vi "校准中 (子VI).vi"(10 "校准按钮":refnum<vi>, 11 "曲线模型":refnum<vi>) -> ()   [LabVIEW 2016, in "斯坦道CODMn新电路板.lvlib"]
uses:
  <vilib>/ptbypt/NI_PtbyPt.lvlib
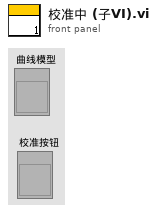
[diagram p1: front panel]
types:
  T1 = enum8{"Enabled", "Disabled", "Disabled and Grayed Out"}
  T2 = cluster{"时间标识":timestamp, "设备":string, "日志信息":string, "流程参数":string}
  T3 = cluster{"系统时间":timestamp, "工作状态":enum16{"空闲", "水样测试", "标样核查", "零点核查", "跨度核查", "空白测试", "平行样测试", "加标回收", "空白校准", "标样校准", "初始化（清洗）"}, "测量模式":enum16{"待机", "连续模式", "周期模式", "定点模式", "受控模式", "手动模式"}, "告警代码":u16, "故障代码":u16, "日志代码":u16, "软件版本":u16, "A":sgl, "B":sgl, "K":sgl, "当前滴定数":sgl, "T":sgl, "H":sgl, "id":u16, "flowid":u16, "量程":u16, "加热实时温度":sgl, "当前ORP值":sgl, "运行时间":sgl, "当前步骤剩余时间":sgl, "结束滴定数":sgl}
  T4 = enum16{"空闲", "水样测试", "标样核查", "零点核查", "跨度核查", "空白测试", "平行样测试", "加标回收", "空白校准", "标样校准", "初始化（清洗）"}
  T5 = cluster{"公式":cluster{"X^2":dbl, "X":dbl, "B":dbl}, "校准":cluster{"校准？":bool, "校准点1-5":u16, "校准浓度":dbl}}
  T6 = cluster{"标液浓度1":dbl, "测量吸光度1":dbl, "样品1启用":bool, "标液浓度2":dbl, "测量吸光度2":dbl, "样品2启用":bool, "标液浓度3":dbl, "测量吸光度3":dbl, "样品3启用":bool, "标液浓度4":dbl, "测量吸光度4":dbl, "样品4启用":bool, "标液浓度5":dbl, "测量吸光度5":dbl, "样品5启用":bool, "模型":enum32{"线性", "多项式"}, "method":enum16{"最小二乘", "最小绝对残差", "Bisquare"}, "精度":dbl, "XY图":cluster{"X Values":dbl[], "Y Values":dbl[]}[], "拟合公式":string, "r^2":dbl}
  T7 = cluster{"测量量程":dbl, "测量精度":dbl, "测量间隔":dbl, "消解温度":dbl, "消解时长":dbl, "空白校准时间":timestamp, "曲线截距":dbl, "曲线斜率":dbl, "测量检出限":dbl, "测量信号值":dbl, "线性相关系数":dbl, "二次多项式系数":dbl, "标样校准时间":timestamp, "稀释倍数":dbl, "三项式系数":dbl, "空白标定系数":dbl, "量程系数":dbl, "F0/ORPA":dbl, "F1/ORPB":dbl, "F2/ORPK":dbl, "F3":dbl, "F4":dbl, "F5":dbl, "F6":dbl, "F7":dbl, "X0/滴定数":dbl, "量程":dbl}
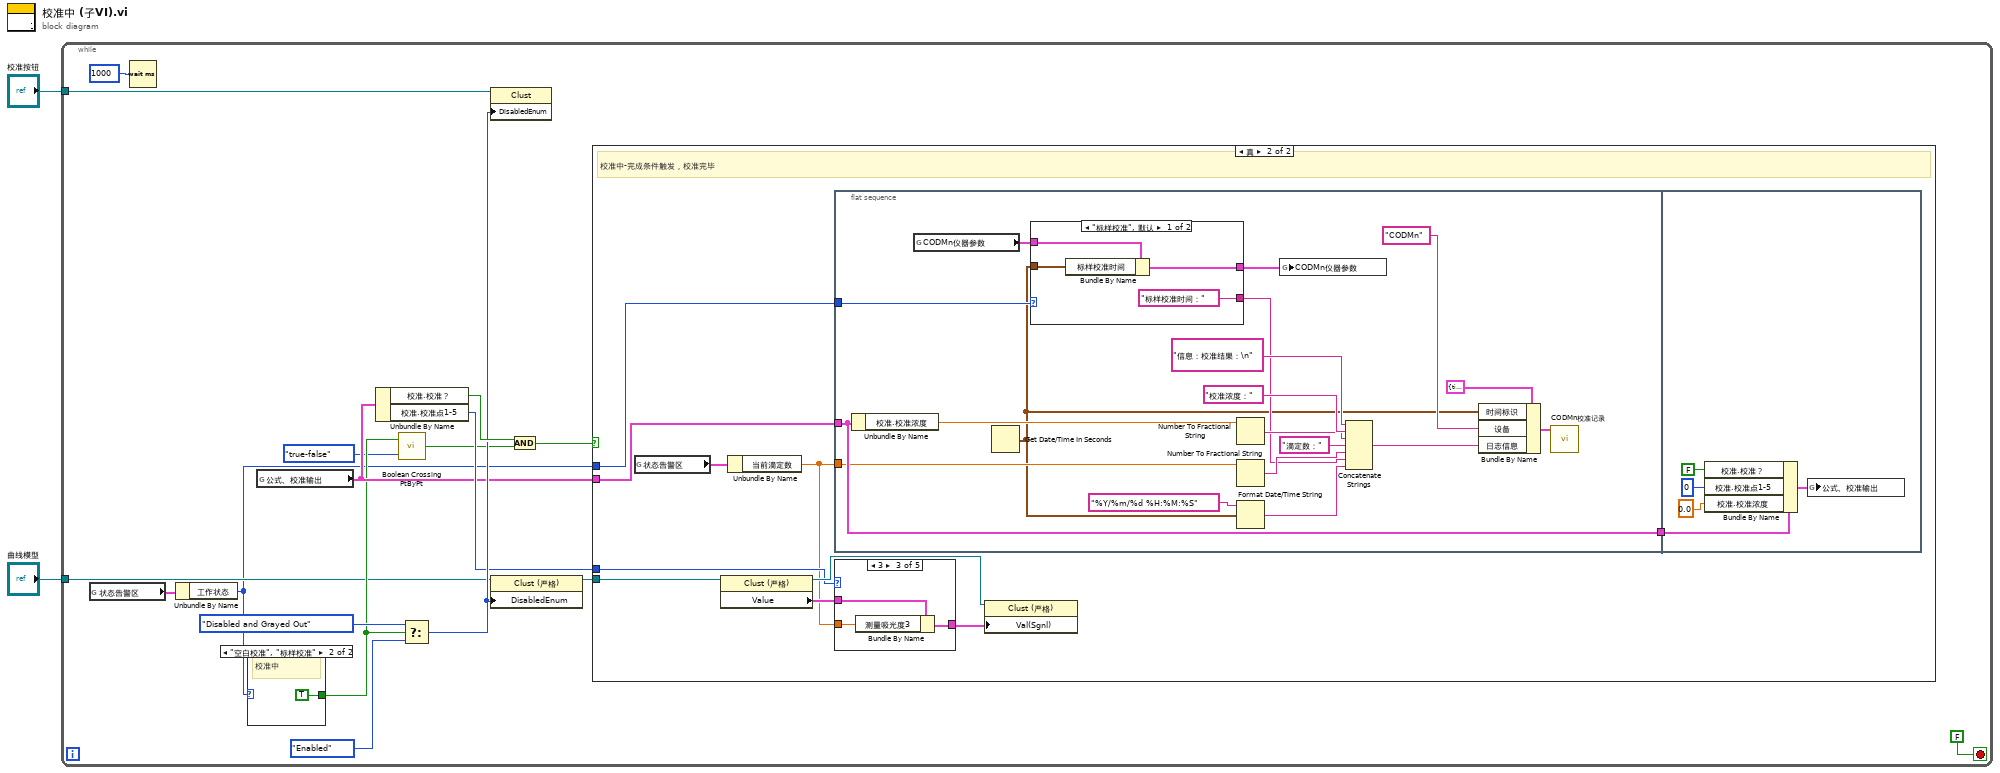
[diagram p0: block diagram]
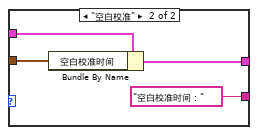
[diagram p3: hidden frame]
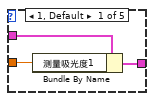
[diagram p4: hidden frame]
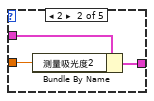
[diagram p5: hidden frame]
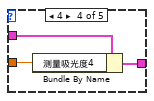
[diagram p6: hidden frame]
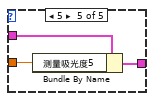
[diagram p7: hidden frame]
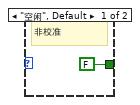
[diagram p8: hidden frame]
diagram:
  n1 = while {
    tunnel: "校准按钮" -> [w5]
    tunnel: "曲线模型" -> [w4]
    stop <- FALSE stop-if-true
    n2 = global read "VARCODMn全局变量.vi" "状态告警区"() -> (w19:T3)
    n3 = Wait (ms)(milliseconds to wait=u32 1000 ("等待时间（毫秒）")) -> ()  [unwired: 1 out]
    n4 = Unbundle By Name(w19) -> ("工作状态"=w3:T4)
    n5 = case shown="\"空白校准\", \"标样校准\"" w3 {
      tunnel: [FALSE TRUE] -> w8
      frame "空闲", Default {
        # "非校准"
      }
      frame "空白校准", "标样校准" {
        # "校准中"
      }
    }
    n6 = global read "CODMn断电保存全局变量.vi" "公式、校准输出"() -> (w9:T5)
    n7 = Unbundle By Name(w9) -> ("校准.校准？"=w18:bool, "校准.校准点1-5"=w10:u16)
    n8 = call <vilib>:"Boolean Crossing PtByPt.vi"("direction"=enum16{"either", "false-true", "true-false"}."true-false", "input"=w8) -> ("crossing"=w6:bool)  [unwired: 1 in]
    n9 = Select(t=T1."Disabled and Grayed Out" ("禁用"), s=w8, f=T1."Enabled" ("禁用")) -> (s? t:f=w13:T1)
    n10 = property class="Clust"(reference=w5, "DisabledEnum"=w13) -> ()  [unwired: 1 in, 2 out]
    n11 = property class="Clust (严格)"(reference=w4, "DisabledEnum"=w13) -> (reference out=w11:refnum<vi>)  [unwired: 1 in, 1 out]
    n12 = And(x=w18, y=w6) -> (x .and. y?=w12:bool)
    n13 = case shown="真" w12 {
      tunnel: w11 -> [_ w29]
      tunnel: w10 -> [_ w26]
      tunnel: w9 -> [_ w23]
      tunnel: w3 -> [_ w20]
      frame False {
      }
      frame True {
        # "校准中-完成条件触发，校准完毕"
        n14 = global read "VARCODMn全局变量.vi" "状态告警区"() -> (w27:T3)
        n15 = property class="Clust (严格)"(reference=w29) -> (reference out=w28:refnum<vi>, "Value"=w25:T6)  [unwired: 1 in, 1 out]
        n16 = Unbundle By Name(w27) -> ("当前滴定数"=w21:sgl)
        n17 = flat-sequence {
          tunnel: w23 -> [w35]
          tunnel: [w35] -> w22
          tunnel: w21 -> [w34]
          tunnel: w20 -> [w33]
          tunnel: w22 -> [w61]
          frame #0 {
            n18 = Unbundle By Name(w35) -> ("校准.校准浓度"=w46:dbl)
            n19 = global read "CODMn断电保存全局变量.vi" "CODMn仪器参数"() -> (w32:T7)
            n20 = Get Date/Time In Seconds() -> (seconds since 1Jan1904=w31:timestamp)
            n21 = case shown="\"标样校准\", 默认" w33 {
              tunnel: ["标样校准时间：" "空白校准时间："] -> w41
              tunnel: w32 -> [w51 w54]
              tunnel: w31 -> [w50 w55]
              tunnel: [w49 w53] -> w30
              frame "标样校准", Default {
                n22 = Bundle By Name(cluster=w51, "标样校准时间"=w50) -> (w49:T7)
              }
              frame "空白校准" {
                n23 = Bundle By Name(cluster=w54, "空白校准时间"=w55) -> (w53:T7)
              }
            }
            n24 = Number To Fractional String(number=w46) -> (F-format string=w45:string)  [unwired: 3 in]
            n25 = Number To Fractional String(number=w34) -> (F-format string=w43:string)  [unwired: 3 in]
            n26 = Format Date/Time String(time format string (%c)="%Y/%m/%d %H:%M:%S" ("时间格式字符串(%c)"), seconds (now)=w31) -> (date/time string=w40:string)  [unwired: 1 in]
            n27 = global write "CODMn断电保存全局变量.vi" "CODMn仪器参数"(w30) -> ()
            n28 = Concatenate Strings("信息：校准结果：\n", "校准浓度：", w45, "滴定数：", w43, w41, w40) -> (w37:string)
            n29 = Bundle By Name(cluster=T2 {"时间标识"=timestamp(0 s since 1904-01-01), "设备"="", "日志信息"="", "流程参数"=""} ("data in"), "时间标识"=w31, "设备"="CODMn", "日志信息"=w37) -> (w36:T2)
            n30 = call "CODMn校准记录.vi"("data in"=w36) -> ()  [unwired: 11 in]
          }
          frame #1 {
            n31 = Bundle By Name(cluster=w61, "校准.校准？"=FALSE, "校准.校准点1-5"=u16 0, "校准.校准浓度"=0.0) -> (w57:T5)
            n32 = global write "CODMn断电保存全局变量.vi" "公式、校准输出"(w57) -> ()
          }
        }
        n33 = case shown="3" w26 {
          tunnel: w25 -> [w64 w67 w70 w73 w75]
          tunnel: [w63 w66 w69 w72 w76] -> w24
          tunnel: w21 -> [w62 w65 w68 w71 w74]
          frame 1, Default {
            n34 = Bundle By Name(cluster=w64, "测量吸光度1"=w62) -> (w63:T6)
          }
          frame 2 {
            n35 = Bundle By Name(cluster=w67, "测量吸光度2"=w65) -> (w66:T6)
          }
          frame 3 {
            n36 = Bundle By Name(cluster=w70, "测量吸光度3"=w68) -> (w69:T6)
          }
          frame 4 {
            n37 = Bundle By Name(cluster=w73, "测量吸光度4"=w71) -> (w72:T6)
          }
          frame 5 {
            n38 = Bundle By Name(cluster=w75, "测量吸光度5"=w74) -> (w76:T6)
          }
        }
        n39 = property class="Clust (严格)"(reference=w28, "Val(Sgnl)"=w24) -> ()  [unwired: 1 in, 2 out]
      }
    }
  }
